vi "AlGaInPAs_v18.vi"(2 "Debug Mode":bool, 3 "Elapsed Time(s)":dbl, 4 "State":enum16{"Edit", "Start", "Run", "End", "Idle"}(ring), 5 "Argument List In":string[](array[string])) -> (0 "Status Out":string, 1 "Argument List Out":string[](array[string]))   [LabVIEW 2011]
panel:
  out "Prep-P liq var":bool
  out "P liq?":bool
  in  "Prep P liq":bool caption="Pre-run"
  in  "P Liq Flow":dbl caption="P bubbler Flow (0-100 sccm)" format="%.2f"
  in  "Run P Liq":bool caption="Run"
  out "GAMFC3 var":dbl=100.0 caption="R3 (0-1000 sscm)" format="%.1f"
  out "GAMFC2 var":dbl=10.0 caption="R2 (0-100 sscm)" format="%.2f"
  out "GAMFC1 var":dbl=1.0 caption="R1 (0-10 sscm)" format="%.2f"
  out "Ga Flow var":dbl=1.0 caption="Ga Flow (0-10 sscm)" format="%.4f"
  out "Prep-In var":bool
  out "Prep-Ga var":bool
  out "Prep-Al var":bool
  out "Prep-P gas var":bool
  out "Prep-As gas var":bool
  out "prep_done":bool
  out "run started":bool
  out "first":bool=TRUE
  out "total time":dbl
  out "is OK?":bool
  out "AsH3?":bool
  out "PH3?":bool
  out "In?":bool
  out "Ga?":bool
  out "Al?":bool
  in  "Prep As gas":bool caption="Pre-run"
  in  "Prep P gas":bool caption="Pre-run"
  in  "Prep In":bool caption="Pre-run"
  in  "prep_time":dbl caption="pre-run time (s)"
  in  "Prep Al":bool caption="Pre-run"
  in  "Run As gas":bool caption="Run"
  in  "As gas Flow":dbl caption="AsH3 Flow (0-10 sccm)" format="%.2f"
  in  "P gas Flow":dbl caption="PH3 Flow (0-100 sccm)" format="%.2f"
  in  "Run P gas":bool caption="Run"
  in  "In Flow":dbl caption="In Flow (0-100 sscm)" format="%.2f"
  in  "Run In":bool caption="Run"
  in  "Run Al":bool caption="Run"
  in  "Al Flow":dbl caption="Al Flow (0-100 sscm)" format="%.2f"
  in  "Cancel":bool
  in  "OK":bool
  out "tTotal(s) 2":dbl
  in  "Ga Tab Control":enum32{"Page 1", "Page 2", "Page 3"}(tab)
  in  "Ga Dilution":bool caption="Dilute"
  in  "Run Ga":bool caption="Run"
  in  "Prep Ga":bool caption="Pre-run"
  out "Ga Flow val":dbl=1.0 caption="Ga Flow (0-10 sscm)" format="%.4f"
  in  "Ga Flow set":dbl=1.0 caption="Ga Flow (0-10 sscm)" format="%.4f"
  out "GAMFC1 val":dbl=1.0 caption="R1 (0-10 sscm)" format="%.4f"
  out "GAMFC3 val":dbl=100.0 caption="R3 (0-1000 sscm)" format="%.1f"
  out "GAMFC2 val":dbl=10.0 caption="R2 (0-100 sscm)" format="%.2f"
  in  "GAMFC1 set":dbl=1.0 caption="R1 (0-10 sscm)" format="%.2f"
  in  "GAMFC2 set":dbl=10.0 caption="R2 (0-100 sscm)" format="%.2f"
  in  "GAMFC3 set":dbl=100.0 caption="R3 (0-1000 sscm)" format="%.1f"
  in  "Ga Calculated":u16(ring)=1 caption="Calculated" items=["Ga flow", "MFC1", "MFC2", "MFC3"]
  # "Add pre-run time to run time in editor."
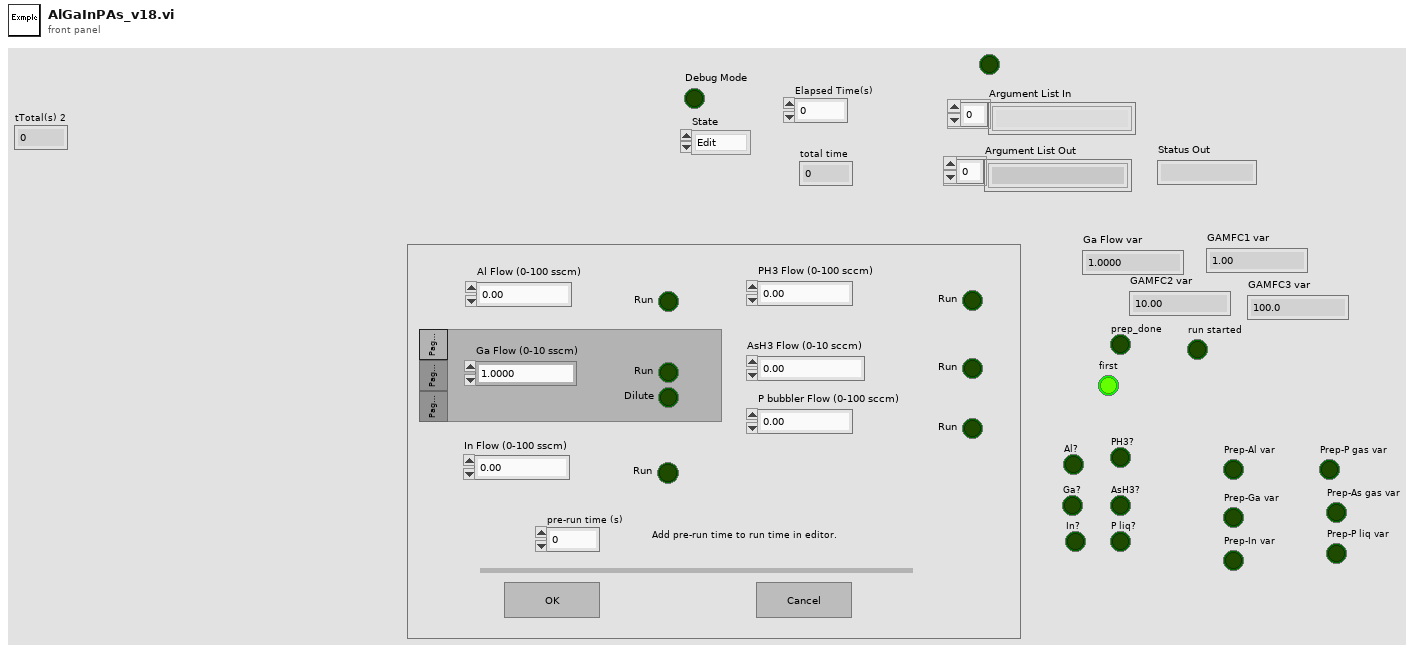
[diagram p1: front panel]
types:
  T1 = enum16{"Discrete", "Continuous", "Instantaneous", "Finite"}
  T2 = enum32{"Invalid", "Default", "Floating", "Floating/Auto-Hide", "Modal"}
  T3 = cluster{"Ga val":bool, "MFC1 val":bool, "MFC2 val":bool, "MFC3 val":bool, "Ga set":bool, "MFC1 set":bool, "MFC2 set":bool, "MFC3 set":bool}
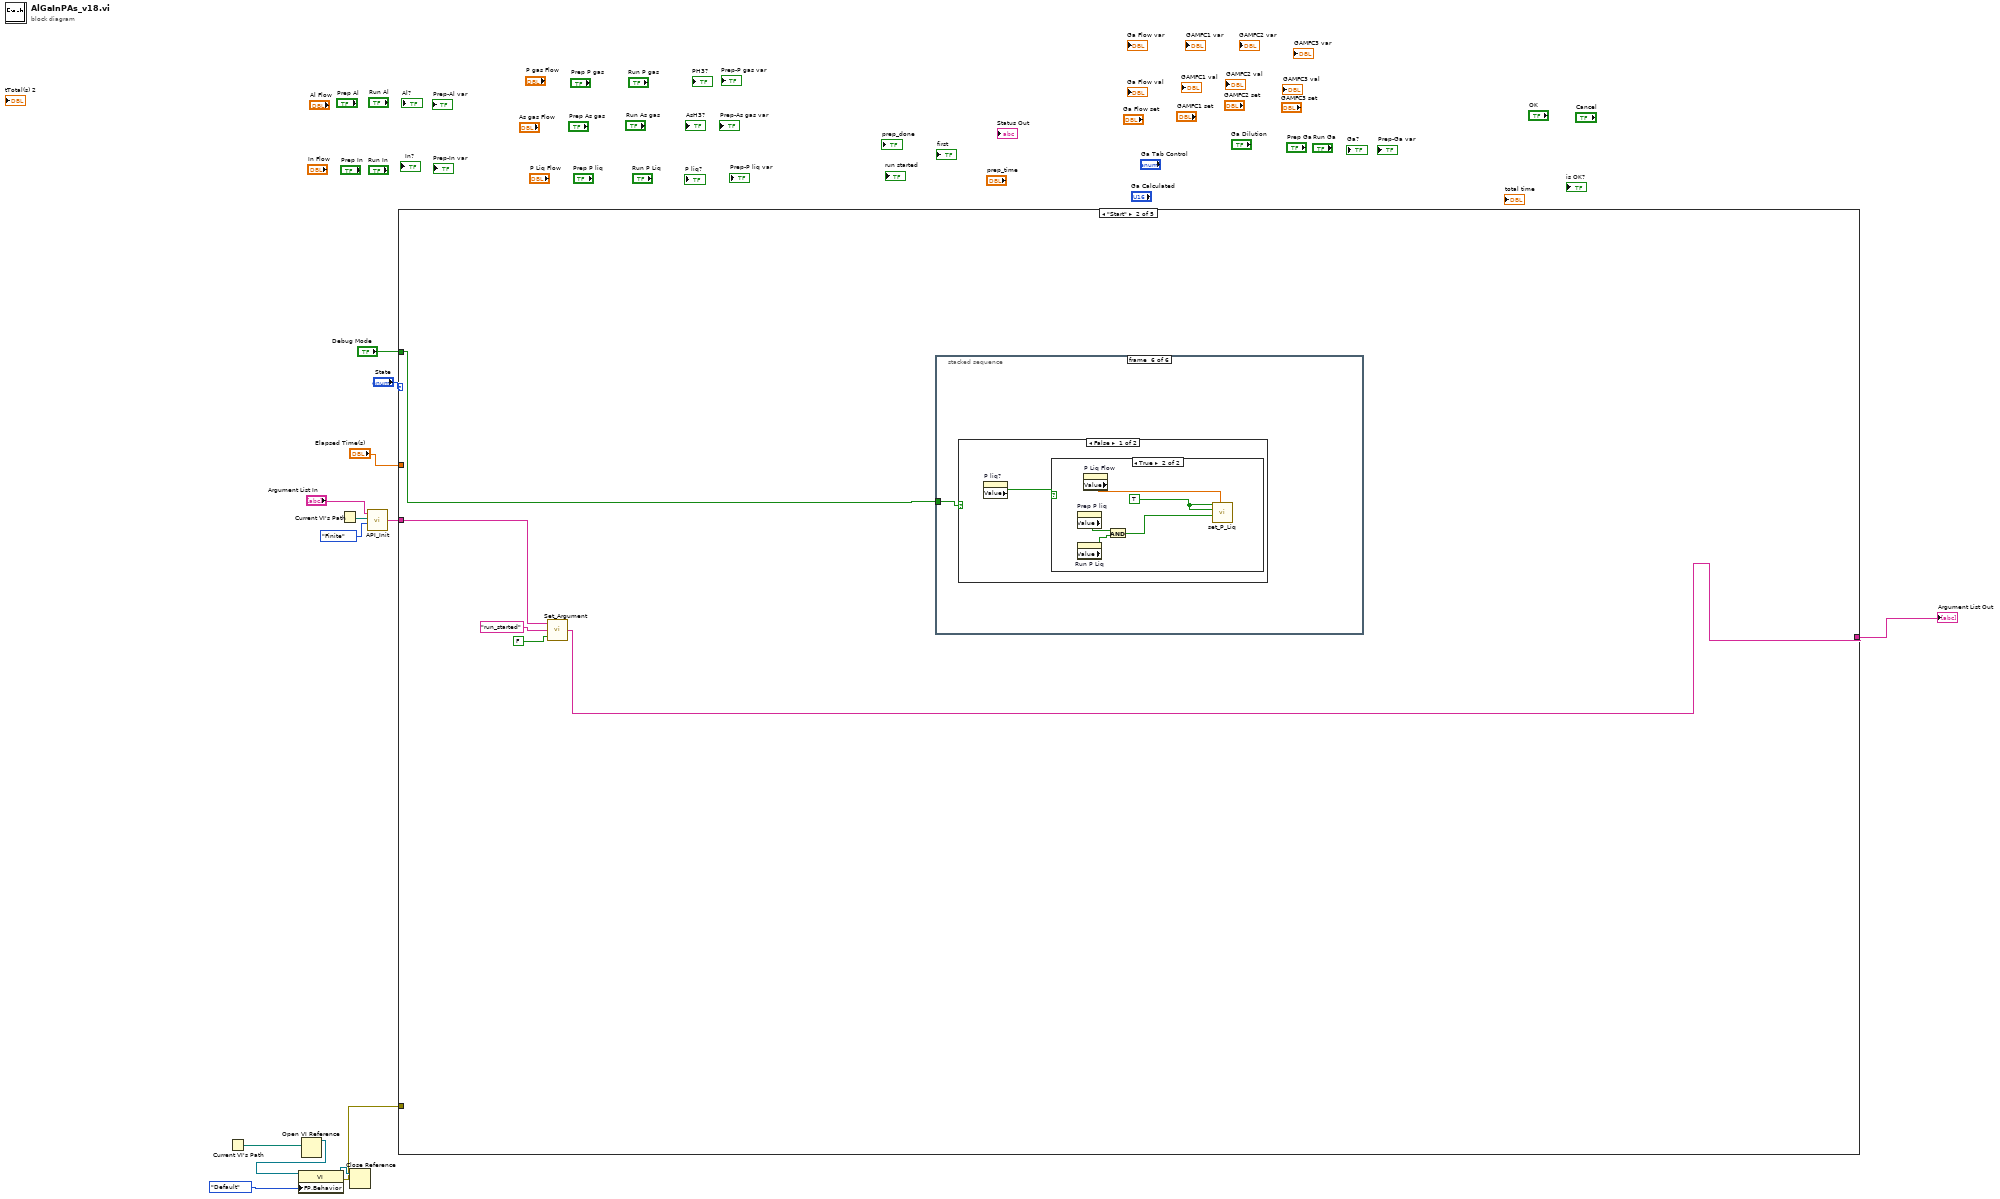
[diagram p0: block diagram]
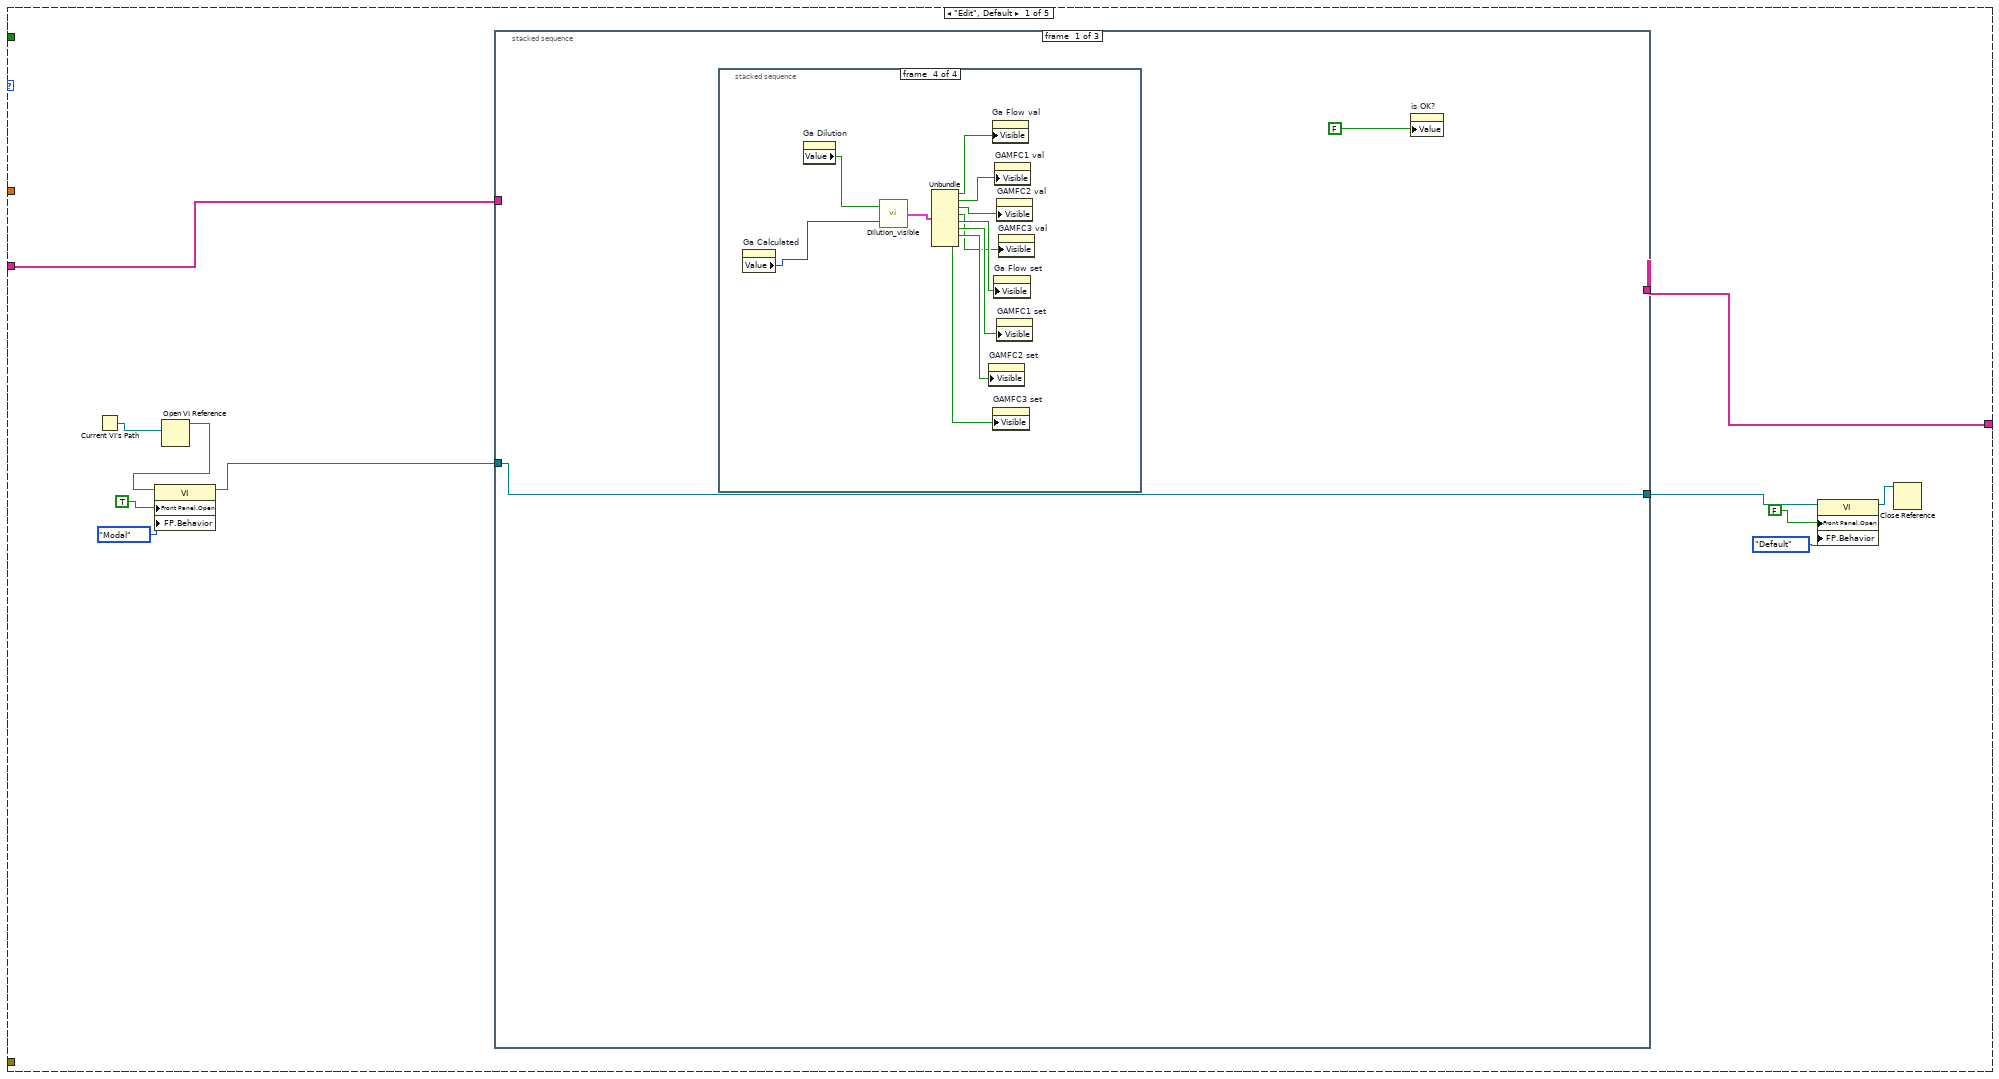
[diagram p2: hidden frame]
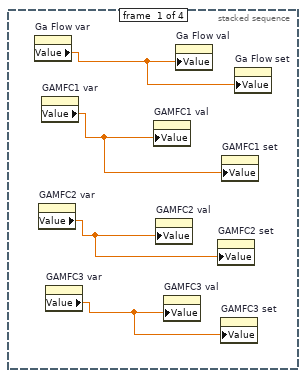
[diagram p3: hidden frame]
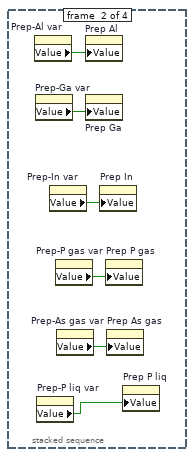
[diagram p4: hidden frame]
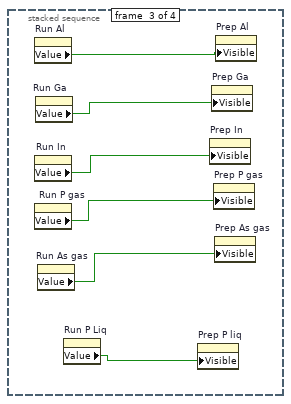
[diagram p5: hidden frame]
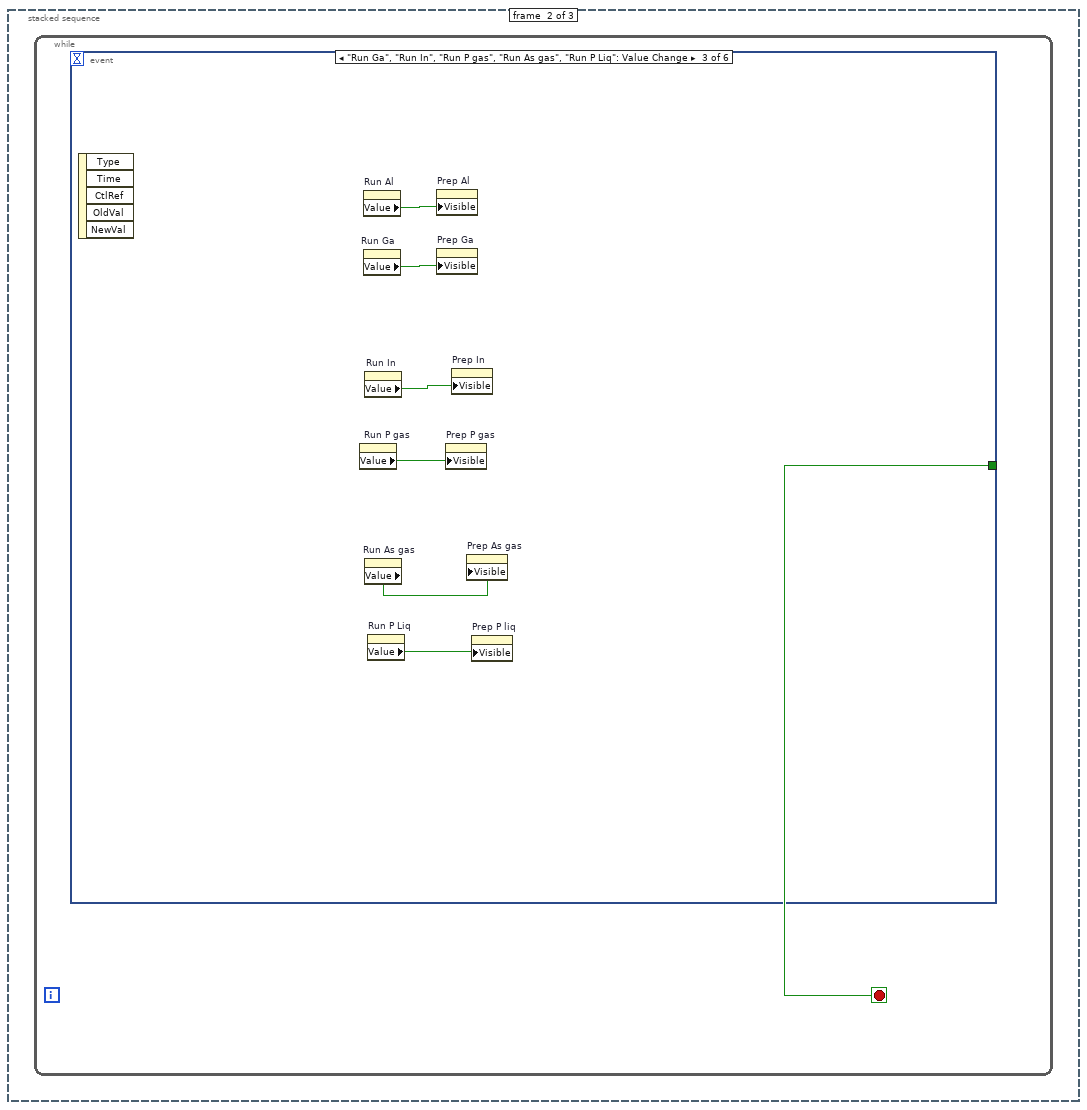
[diagram p6: hidden frame]
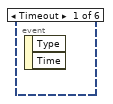
[diagram p7: hidden frame]
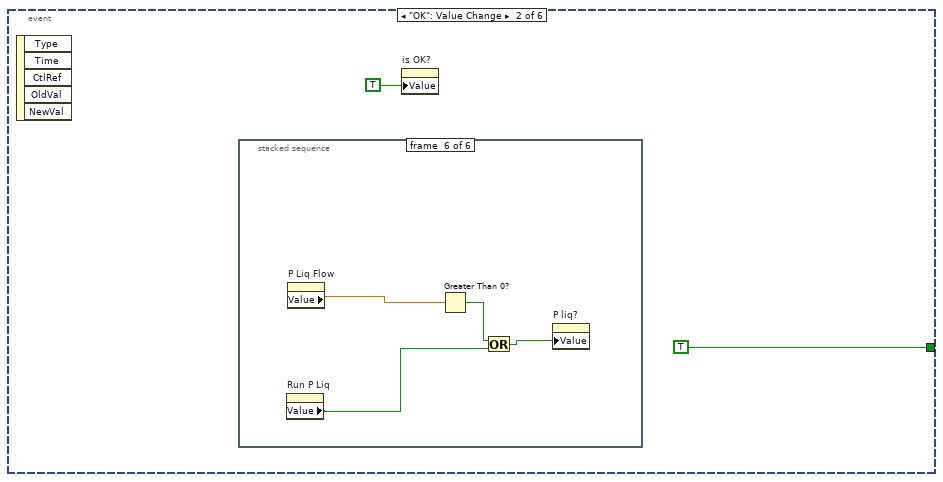
[diagram p8: hidden frame]
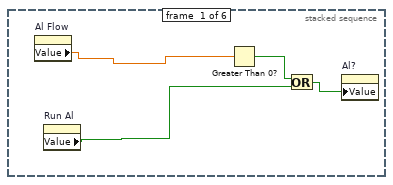
[diagram p9: hidden frame]
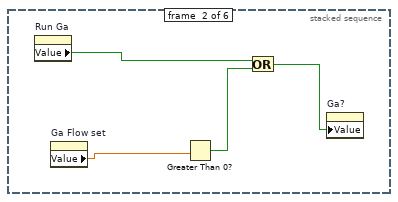
[diagram p10: hidden frame]
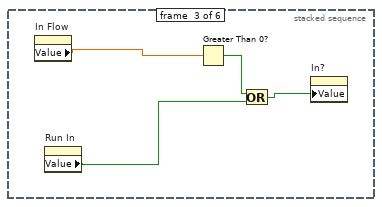
[diagram p11: hidden frame]
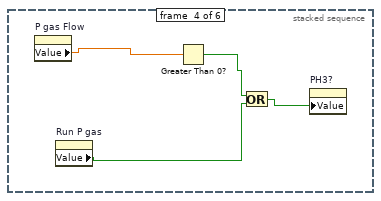
[diagram p12: hidden frame]
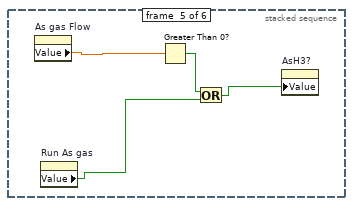
[diagram p13: hidden frame]
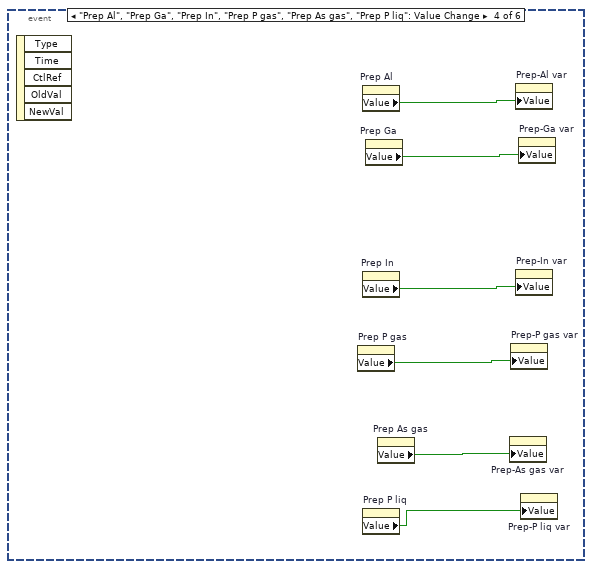
[diagram p14: hidden frame]
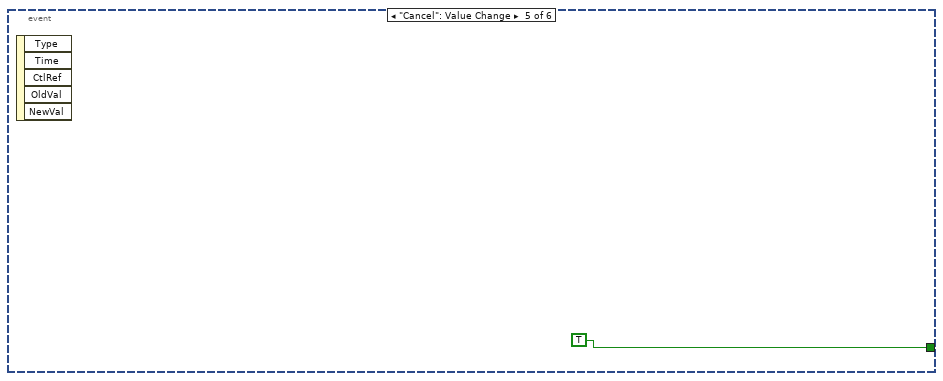
[diagram p15: hidden frame]
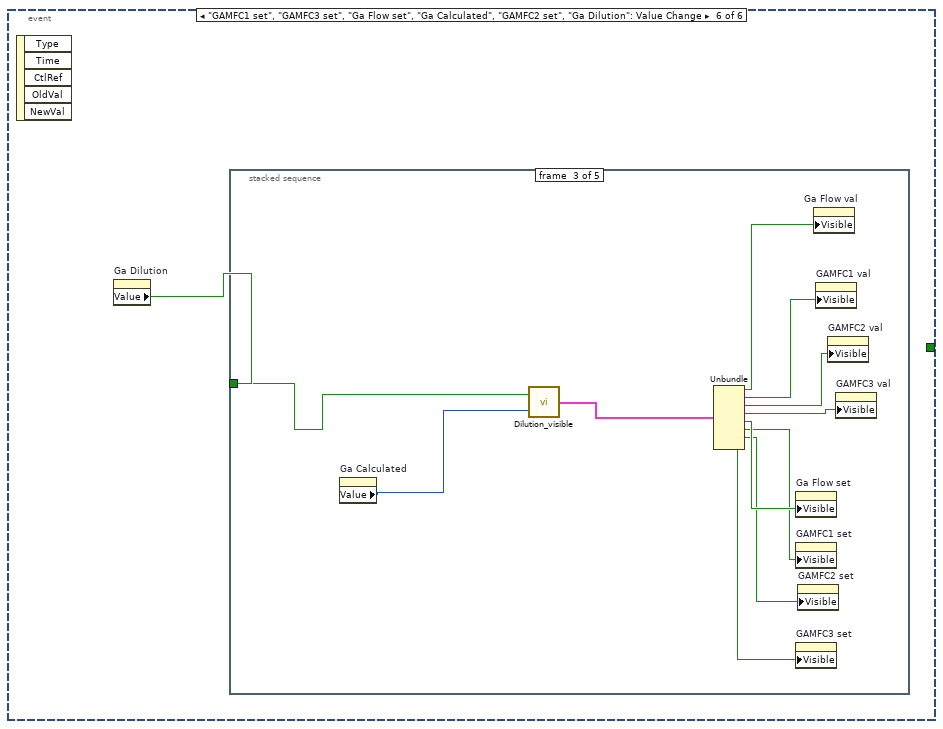
[diagram p16: hidden frame]
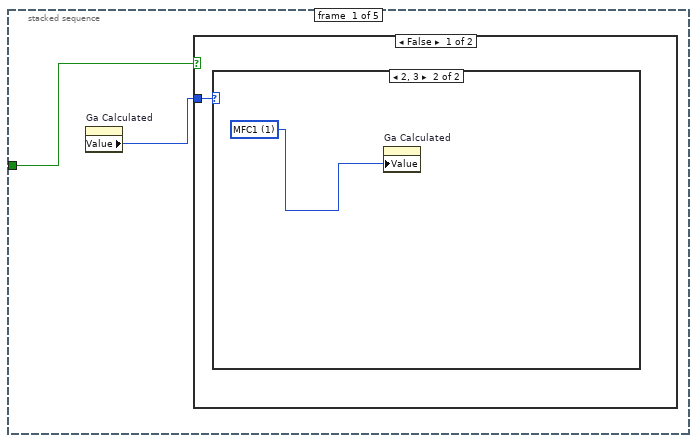
[diagram p17: hidden frame]
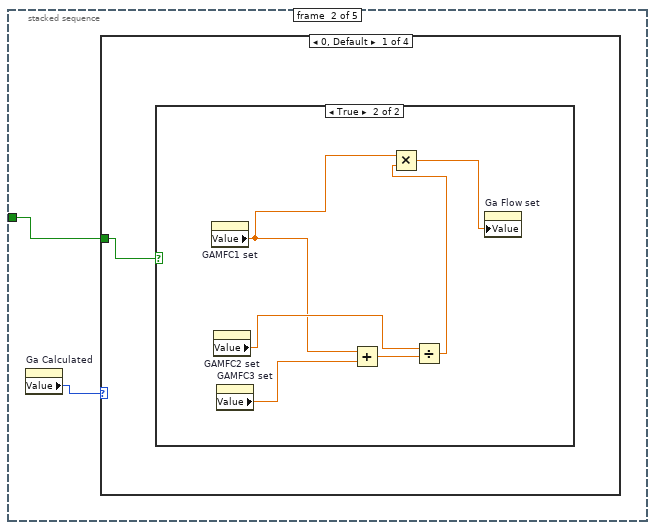
[diagram p20: hidden frame]
diagram:
  n1 = Current VI's Path() -> (path=w9:path)
  n2 = Open VI Reference(vi path=w9) -> (vi reference=w8:refnum<vi>)  [unwired: 1 in, 5 out]
  n3 = property class="VI"(reference=w8, "FP.Behavior"=T2."Default" ("Front Panel Window:Behavior")) -> (reference out=w6:refnum<vi>, error out=w5:errorcluster)  [unwired: 1 in]
  n4 = Current VI's Path() -> (path=w4:path)
  n5 = Close Reference(reference=w6) -> ()  [unwired: 1 in, 1 out]
  n6 = call "API_Init.vi"("API Mode"=T1."Finite", "VI Path"=w4, "Argument List In"="Argument List In") -> ("Argument List Out"=w1:string[])  [unwired: 1 in]
  n7 = case shown="\"Start\"" "State" {
    tunnel: "Debug Mode" -> [_ w157 w220 _ _]
    tunnel: "Elapsed Time(s)" -> [_ _ w222 _ _]
    tunnel: w1 -> [w15 w159 w219 w360 w361]
    tunnel: [w14 w158 w221 w360 w361] -> w10
    tunnel: w5 -> [_ _ _ _ _]
    frame "Edit", Default {
      n8 = Current VI's Path() -> (path=w20:path)
      n9 = Open VI Reference(vi path=w20) -> (vi reference=w19:refnum<vi>)  [unwired: 1 in, 5 out]
      n10 = property class="VI"(reference=w19, "Front Panel.Open"=TRUE ("Front Panel Window:Open"), "FP.Behavior"=T2."Modal" ("Front Panel Window:Behavior")) -> (reference out=w18:refnum<vi>)  [unwired: 1 in, 1 out]
      n11 = stacked-sequence {
        tunnel: w15 -> [_ _ w152]
        tunnel: w18 -> [w26 _ _]
        tunnel: [w26 _ _] -> w22
        tunnel: [_ _ w150] -> w14
        frame #0 {
          n12 = stacked-sequence {
            frame #0 {
              n13 = property on="Ga Flow var" class="DigNum (strict)"() -> ("Value"=w30:dbl)  [unwired: 2 in, 2 out]
              n14 = property on="GAMFC2 var" class="DigNum (strict)"() -> ("Value"=w28:dbl)  [unwired: 2 in, 2 out]
              n15 = property on="GAMFC1 var" class="DigNum (strict)"() -> ("Value"=w27:dbl)  [unwired: 2 in, 2 out]
              n16 = property on="GAMFC3 var" class="DigNum (strict)"() -> ("Value"=w29:dbl)  [unwired: 2 in, 2 out]
              n17 = property on="GAMFC1 val" class="DigNum (strict)"("Value"=w27) -> ()  [unwired: 2 in, 2 out]
              n18 = property on="GAMFC2 val" class="DigNum (strict)"("Value"=w28) -> ()  [unwired: 2 in, 2 out]
              n19 = property on="GAMFC3 val" class="DigNum (strict)"("Value"=w29) -> ()  [unwired: 2 in, 2 out]
              n20 = property on="Ga Flow val" class="DigNum (strict)"("Value"=w30) -> ()  [unwired: 2 in, 2 out]
              n21 = property on="GAMFC2 set" class="DigNum (strict)"("Value"=w28) -> ()  [unwired: 2 in, 2 out]
              n22 = property on="GAMFC3 set" class="DigNum (strict)"("Value"=w29) -> ()  [unwired: 2 in, 2 out]
              n23 = property on="GAMFC1 set" class="DigNum (strict)"("Value"=w27) -> ()  [unwired: 2 in, 2 out]
              n24 = property on="Ga Flow set" class="DigNum (strict)"("Value"=w30) -> ()  [unwired: 2 in, 2 out]
            }
            frame #1 {
              n25 = property on="Prep-Al var" class="Bool (strict)"() -> ("Value"=w36:bool)  [unwired: 2 in, 2 out]
              n26 = property on="Prep-Ga var" class="Bool (strict)"() -> ("Value"=w35:bool)  [unwired: 2 in, 2 out]
              n27 = property on="Prep-P liq var" class="Bool (strict)"() -> ("Value"=w31:bool)  [unwired: 2 in, 2 out]
              n28 = property on="Prep-In var" class="Bool (strict)"() -> ("Value"=w34:bool)  [unwired: 2 in, 2 out]
              n29 = property on="Prep-P gas var" class="Bool (strict)"() -> ("Value"=w33:bool)  [unwired: 2 in, 2 out]
              n30 = property on="Prep-As gas var" class="Bool (strict)"() -> ("Value"=w32:bool)  [unwired: 2 in, 2 out]
              n31 = property on="Prep Al" class="Bool (strict)"("Value"=w36) -> ()  [unwired: 2 in, 2 out]
              n32 = property on="Prep Ga" class="Bool (strict)"("Value"=w35) -> ()  [unwired: 2 in, 2 out]
              n33 = property on="Prep In" class="Bool (strict)"("Value"=w34) -> ()  [unwired: 2 in, 2 out]
              n34 = property on="Prep P gas" class="Bool (strict)"("Value"=w33) -> ()  [unwired: 2 in, 2 out]
              n35 = property on="Prep As gas" class="Bool (strict)"("Value"=w32) -> ()  [unwired: 2 in, 2 out]
              n36 = property on="Prep P liq" class="Bool (strict)"("Value"=w31) -> ()  [unwired: 2 in, 2 out]
            }
            frame #2 {
              n37 = property on="Run Al" class="Bool (strict)"() -> ("Value"=w42:bool)  [unwired: 2 in, 2 out]
              n38 = property on="Run In" class="Bool (strict)"() -> ("Value"=w40:bool)  [unwired: 2 in, 2 out]
              n39 = property on="Run P gas" class="Bool (strict)"() -> ("Value"=w39:bool)  [unwired: 2 in, 2 out]
              n40 = property on="Run Ga" class="Bool (strict)"() -> ("Value"=w41:bool)  [unwired: 2 in, 2 out]
              n41 = property on="Run As gas" class="Bool (strict)"() -> ("Value"=w38:bool)  [unwired: 2 in, 2 out]
              n42 = property on="Run P Liq" class="Bool (strict)"() -> ("Value"=w37:bool)  [unwired: 2 in, 2 out]
              n43 = property on="Prep P liq" class="Bool (strict)"("Visible"=w37) -> ()  [unwired: 2 in, 2 out]
              n44 = property on="Prep In" class="Bool (strict)"("Visible"=w40) -> ()  [unwired: 2 in, 2 out]
              n45 = property on="Prep Ga" class="Bool (strict)"("Visible"=w41) -> ()  [unwired: 2 in, 2 out]
              n46 = property on="Prep P gas" class="Bool (strict)"("Visible"=w39) -> ()  [unwired: 2 in, 2 out]
              n47 = property on="Prep As gas" class="Bool (strict)"("Visible"=w38) -> ()  [unwired: 2 in, 2 out]
              n48 = property on="Prep Al" class="Bool (strict)"("Visible"=w42) -> ()  [unwired: 2 in, 2 out]
            }
            frame #3 {
              n49 = property on="Ga Calculated" class="Ring (strict)"() -> ("Value"=w43:u16)  [unwired: 2 in, 2 out]
              n50 = property on="Ga Dilution" class="Bool (strict)"() -> ("Value"=w53:bool)  [unwired: 2 in, 2 out]
              n51 = call "Dilution_visible.vi"("calculated"=w43, "dilution"=w53) -> ("Visible"=w45:T3)
              n52 = Unbundle(w45) -> ("Ga val"=w46:bool, "MFC1 val"=w47:bool, "MFC2 val"=w44:bool, "MFC3 val"=w48:bool, "Ga set"=w49:bool, "MFC1 set"=w50:bool, "MFC2 set"=w51:bool, "MFC3 set"=w52:bool)
              n53 = property on="GAMFC2 set" class="DigNum (strict)"("Visible"=w51) -> ()  [unwired: 2 in, 2 out]
              n54 = property on="Ga Flow val" class="DigNum (strict)"("Visible"=w46) -> ()  [unwired: 2 in, 2 out]
              n55 = property on="GAMFC3 set" class="DigNum (strict)"("Visible"=w52) -> ()  [unwired: 2 in, 2 out]
              n56 = property on="Ga Flow set" class="DigNum (strict)"("Visible"=w49) -> ()  [unwired: 2 in, 2 out]
              n57 = property on="GAMFC1 val" class="DigNum (strict)"("Visible"=w47) -> ()  [unwired: 2 in, 2 out]
              n58 = property on="GAMFC2 val" class="DigNum (strict)"("Visible"=w44) -> ()  [unwired: 2 in, 2 out]
              n59 = property on="GAMFC1 set" class="DigNum (strict)"("Visible"=w50) -> ()  [unwired: 2 in, 2 out]
              n60 = property on="GAMFC3 val" class="DigNum (strict)"("Visible"=w48) -> ()  [unwired: 2 in, 2 out]
            }
          }
          n61 = property on="is OK?" class="Bool (strict)"("Value"=FALSE ("is OK?")) -> ()  [unwired: 2 in, 2 out]
        }
        frame #1 {
          n62 = while {
            stop <- w54 stop-if-true
            n63 = event shown="[2] \"Run Ga\", \"Run In\", \"Run P gas\", \"Run As gas\", \"Run P Liq\": Value Change" {
              selector: _ -> [_ _ _ _ _ _]
              dyn-events: _ -> [_ _ _ _ _ _]
              timeout: _ -> [_ _ _ _ _ _]
              tunnel: [_ TRUE _ _ TRUE _] -> w54
              event Timeout {
                n64 = event-data() -> ()  [unwired: 1 in, 2 out]
              }
              event "OK": Value Change {
                n65 = event-data() -> ()  [unwired: 1 in, 5 out]
                n66 = stacked-sequence {
                  frame #0 {
                    n67 = property on="Al Flow" class="DigNum (strict)"() -> ("Value"=w59:dbl)  [unwired: 2 in, 2 out]
                    n68 = property on="Run Al" class="Bool (strict)"() -> ("Value"=w58:bool)  [unwired: 2 in, 2 out]
                    n69 = Greater Than 0?(x=w59) -> (x > 0?=w60:bool)
                    n70 = Or(x=w60, y=w58) -> (x .or. y?=w57:bool)
                    n71 = property on="Al?" class="Bool (strict)"("Value"=w57) -> ()  [unwired: 2 in, 2 out]
                  }
                  frame #1 {
                    n72 = property on="Run Ga" class="Bool (strict)"() -> ("Value"=w62:bool)  [unwired: 2 in, 2 out]
                    n73 = property on="Ga Flow set" class="DigNum (strict)"() -> ("Value"=w63:dbl)  [unwired: 2 in, 2 out]
                    n74 = Greater Than 0?(x=w63) -> (x > 0?=w64:bool)
                    n75 = Or(x=w62, y=w64) -> (x .or. y?=w61:bool)
                    n76 = property on="Ga?" class="Bool (strict)"("Value"=w61) -> ()  [unwired: 2 in, 2 out]
                  }
                  frame #2 {
                    n77 = property on="In Flow" class="DigNum (strict)"() -> ("Value"=w66:dbl)  [unwired: 2 in, 2 out]
                    n78 = property on="Run In" class="Bool (strict)"() -> ("Value"=w67:bool)  [unwired: 2 in, 2 out]
                    n79 = Greater Than 0?(x=w66) -> (x > 0?=w68:bool)
                    n80 = Or(x=w68, y=w67) -> (x .or. y?=w65:bool)
                    n81 = property on="In?" class="Bool (strict)"("Value"=w65) -> ()  [unwired: 2 in, 2 out]
                  }
                  frame #3 {
                    n82 = property on="P gas Flow" class="DigNum (strict)"() -> ("Value"=w71:dbl)  [unwired: 2 in, 2 out]
                    n83 = property on="Run P gas" class="Bool (strict)"() -> ("Value"=w70:bool)  [unwired: 2 in, 2 out]
                    n84 = Greater Than 0?(x=w71) -> (x > 0?=w72:bool)
                    n85 = Or(x=w72, y=w70) -> (x .or. y?=w69:bool)
                    n86 = property on="PH3?" class="Bool (strict)"("Value"=w69) -> ()  [unwired: 2 in, 2 out]
                  }
                  frame #4 {
                    n87 = property on="As gas Flow" class="DigNum (strict)"() -> ("Value"=w75:dbl)  [unwired: 2 in, 2 out]
                    n88 = property on="Run As gas" class="Bool (strict)"() -> ("Value"=w74:bool)  [unwired: 2 in, 2 out]
                    n89 = Greater Than 0?(x=w75) -> (x > 0?=w76:bool)
                    n90 = Or(x=w76, y=w74) -> (x .or. y?=w73:bool)
                    n91 = property on="AsH3?" class="Bool (strict)"("Value"=w73) -> ()  [unwired: 2 in, 2 out]
                  }
                  frame #5 {
                    n92 = property on="Run P Liq" class="Bool (strict)"() -> ("Value"=w79:bool)  [unwired: 2 in, 2 out]
                    n93 = property on="P Liq Flow" class="DigNum (strict)"() -> ("Value"=w78:dbl)  [unwired: 2 in, 2 out]
                    n94 = Greater Than 0?(x=w78) -> (x > 0?=w80:bool)
                    n95 = Or(x=w80, y=w79) -> (x .or. y?=w77:bool)
                    n96 = property on="P liq?" class="Bool (strict)"("Value"=w77) -> ()  [unwired: 2 in, 2 out]
                  }
                }
                n97 = property on="is OK?" class="Bool (strict)"("Value"=TRUE ("is OK?")) -> ()  [unwired: 2 in, 2 out]
              }
              event "Run Ga", "Run In", "Run P gas", "Run As gas", "Run P Liq": Value Change {
                n98 = event-data() -> ()  [unwired: 1 in, 5 out]
                n99 = property on="Run P gas" class="Bool (strict)"() -> ("Value"=w82:bool)  [unwired: 2 in, 2 out]
                n100 = property on="Run Al" class="Bool (strict)"() -> ("Value"=w86:bool)  [unwired: 2 in, 2 out]
                n101 = property on="Run Ga" class="Bool (strict)"() -> ("Value"=w85:bool)  [unwired: 2 in, 2 out]
                n102 = property on="Run In" class="Bool (strict)"() -> ("Value"=w84:bool)  [unwired: 2 in, 2 out]
                n103 = property on="Run As gas" class="Bool (strict)"() -> ("Value"=w83:bool)  [unwired: 2 in, 2 out]
                n104 = property on="Run P Liq" class="Bool (strict)"() -> ("Value"=w81:bool)  [unwired: 2 in, 2 out]
                n105 = property on="Prep Al" class="Bool (strict)"("Visible"=w86) -> ()  [unwired: 2 in, 2 out]
                n106 = property on="Prep Ga" class="Bool (strict)"("Visible"=w85) -> ()  [unwired: 2 in, 2 out]
                n107 = property on="Prep P gas" class="Bool (strict)"("Visible"=w82) -> ()  [unwired: 2 in, 2 out]
                n108 = property on="Prep In" class="Bool (strict)"("Visible"=w84) -> ()  [unwired: 2 in, 2 out]
                n109 = property on="Prep As gas" class="Bool (strict)"("Visible"=w83) -> ()  [unwired: 2 in, 2 out]
                n110 = property on="Prep P liq" class="Bool (strict)"("Visible"=w81) -> ()  [unwired: 2 in, 2 out]
              }
              event "Prep Al", "Prep Ga", "Prep In", "Prep P gas", "Prep As gas", "Prep P liq": Value Change {
                n111 = event-data() -> ()  [unwired: 1 in, 5 out]
                n112 = property on="Prep P gas" class="Bool (strict)"() -> ("Value"=w89:bool)  [unwired: 2 in, 2 out]
                n113 = property on="Prep Al" class="Bool (strict)"() -> ("Value"=w92:bool)  [unwired: 2 in, 2 out]
                n114 = property on="Prep In" class="Bool (strict)"() -> ("Value"=w90:bool)  [unwired: 2 in, 2 out]
                n115 = property on="Prep P liq" class="Bool (strict)"() -> ("Value"=w87:bool)  [unwired: 2 in, 2 out]
                n116 = property on="Prep Ga" class="Bool (strict)"() -> ("Value"=w91:bool)  [unwired: 2 in, 2 out]
                n117 = property on="Prep As gas" class="Bool (strict)"() -> ("Value"=w88:bool)  [unwired: 2 in, 2 out]
                n118 = property on="Prep-As gas var" class="Bool (strict)"("Value"=w88) -> ()  [unwired: 2 in, 2 out]
                n119 = property on="Prep-P gas var" class="Bool (strict)"("Value"=w89) -> ()  [unwired: 2 in, 2 out]
                n120 = property on="Prep-Al var" class="Bool (strict)"("Value"=w92) -> ()  [unwired: 2 in, 2 out]
                n121 = property on="Prep-In var" class="Bool (strict)"("Value"=w90) -> ()  [unwired: 2 in, 2 out]
                n122 = property on="Prep-Ga var" class="Bool (strict)"("Value"=w91) -> ()  [unwired: 2 in, 2 out]
                n123 = property on="Prep-P liq var" class="Bool (strict)"("Value"=w87) -> ()  [unwired: 2 in, 2 out]
              }
              event "Cancel": Value Change {
                n124 = event-data() -> ()  [unwired: 1 in, 5 out]
              }
              event "GAMFC1 set", "GAMFC3 set", "Ga Flow set", "Ga Calculated", "GAMFC2 set", "Ga Dilution": Value Change {
                n125 = event-data() -> ()  [unwired: 1 in, 5 out]
                n126 = property on="Ga Dilution" class="Bool (strict)"() -> ("Value"=w94:bool)  [unwired: 2 in, 2 out]
                n127 = stacked-sequence {
                  tunnel: w94 -> [w96 w100 w141 _ w146]
                  frame #0 {
                    n128 = property on="Ga Calculated" class="Ring (strict)"() -> ("Value"=w95:u16)  [unwired: 2 in, 2 out]
                    n129 = case shown="False" w96 {
                      tunnel: w95 -> [w97 _]
                      frame False {
                        n130 = case shown="2, 3" w97 {
                          frame 0, 1, Default {
                          }
                          frame 2, 3 {
                            w98 = u16 1 items=["Ga flow", "MFC1", "MFC2", "MFC3"] ("Ga calculated")
                            n131 = property on="Ga Calculated" class="Ring (strict)"("Value"=w98) -> ()  [unwired: 2 in, 2 out]
                          }
                        }
                      }
                      frame True {
                      }
                    }
                  }
                  frame #1 {
                    n132 = property on="Ga Calculated" class="Ring (strict)"() -> ("Value"=w99:u16)  [unwired: 2 in, 2 out]
                    n133 = case shown="0, Default" w99 {
                      tunnel: w100 -> [w101 w109 w117 w124]
                      frame 0, Default {
                        n134 = case shown="True" w101 {
                          frame False {
                            n135 = property on="GAMFC1 set" class="DigNum (strict)"() -> ("Value"=w102:dbl)  [unwired: 2 in, 2 out]
                            n136 = property on="Ga Flow set" class="DigNum (strict)"("Value"=w102) -> ()  [unwired: 2 in, 2 out]
                          }
                          frame True {
                            n137 = property on="GAMFC1 set" class="DigNum (strict)"() -> ("Value"=w104:dbl)  [unwired: 2 in, 2 out]
                            n138 = property on="GAMFC2 set" class="DigNum (strict)"() -> ("Value"=w106:dbl)  [unwired: 2 in, 2 out]
                            n139 = property on="GAMFC3 set" class="DigNum (strict)"() -> ("Value"=w108:dbl)  [unwired: 2 in, 2 out]
                            n140 = Add(x=w104, y=w108) -> (x+y=w107:dbl)
                            n141 = Divide(x=w106, y=w107) -> (x/y=w105:dbl)
                            n142 = Multiply(x=w104, y=w105) -> (x*y=w103:dbl)
                            n143 = property on="Ga Flow set" class="DigNum (strict)"("Value"=w103) -> ()  [unwired: 2 in, 2 out]
                          }
                        }
                      }
                      frame 1 {
                        n144 = case shown="True" w109 {
                          frame False {
                            n145 = property on="Ga Flow set" class="DigNum (strict)"() -> ("Value"=w110:dbl)  [unwired: 2 in, 2 out]
                            n146 = property on="GAMFC1 set" class="DigNum (strict)"("Value"=w110) -> ()  [unwired: 2 in, 2 out]
                          }
                          frame True {
                            n147 = property on="Ga Flow set" class="DigNum (strict)"() -> ("Value"=w115:dbl)  [unwired: 2 in, 2 out]
                            n148 = property on="GAMFC2 set" class="DigNum (strict)"() -> ("Value"=w116:dbl)  [unwired: 2 in, 2 out]
                            n149 = property on="GAMFC3 set" class="DigNum (strict)"() -> ("Value"=w114:dbl)  [unwired: 2 in, 2 out]
                            n150 = Subtract(x=w116, y=w115) -> (x-y=w112:dbl)
                            n151 = Multiply(x=w115, y=w114) -> (x*y=w113:dbl)
                            n152 = Divide(x=w113, y=w112) -> (x/y=w111:dbl)
                            n153 = property on="GAMFC1 set" class="DigNum (strict)"("Value"=w111) -> ()  [unwired: 2 in, 2 out]
                          }
                        }
                      }
                      frame 2 {
                        n154 = case shown="True" w117 {
                          frame False {
                          }
                          frame True {
                            n155 = property on="GAMFC1 set" class="DigNum (strict)"() -> ("Value"=w119:dbl)  [unwired: 2 in, 2 out]
                            n156 = property on="GAMFC3 set" class="DigNum (strict)"() -> ("Value"=w121:dbl)  [unwired: 2 in, 2 out]
                            n157 = property on="Ga Flow set" class="DigNum (strict)"() -> ("Value"=w122:dbl)  [unwired: 2 in, 2 out]
                            n158 = Add(x=w119, y=w121) -> (x+y=w123:dbl)
                            n159 = Multiply(x=w122, y=w123) -> (x*y=w120:dbl)
                            n160 = Divide(x=w120, y=w119) -> (x/y=w118:dbl)
                            n161 = property on="GAMFC2 set" class="DigNum (strict)"("Value"=w118) -> ()  [unwired: 2 in, 2 out]
                          }
                        }
                      }
                      frame 3 {
                        n162 = case shown="True" w124 {
                          frame False {
                          }
                          frame True {
                            n163 = property on="GAMFC2 set" class="DigNum (strict)"() -> ("Value"=w130:dbl)  [unwired: 2 in, 2 out]
                            n164 = property on="Ga Flow set" class="DigNum (strict)"() -> ("Value"=w128:dbl)  [unwired: 2 in, 2 out]
                            n165 = property on="GAMFC1 set" class="DigNum (strict)"() -> ("Value"=w129:dbl)  [unwired: 2 in, 2 out]
                            n166 = Subtract(x=w130, y=w128) -> (x-y=w126:dbl)
                            n167 = Divide(x=w129, y=w128) -> (x/y=w127:dbl)
                            n168 = Multiply(x=w127, y=w126) -> (x*y=w125:dbl)
                            n169 = property on="GAMFC3 set" class="DigNum (strict)"("Value"=w125) -> ()  [unwired: 2 in, 2 out]
                          }
                        }
                      }
                    }
                  }
                  frame #2 {
                    n170 = property on="Ga Calculated" class="Ring (strict)"() -> ("Value"=w131:u16)  [unwired: 2 in, 2 out]
                    n171 = call "Dilution_visible.vi"("calculated"=w131, "dilution"=w141) -> ("Visible"=w137:T3)
                    n172 = Unbundle(w137) -> ("Ga val"=w140:bool, "MFC1 val"=w139:bool, "MFC2 val"=w138:bool, "MFC3 val"=w136:bool, "Ga set"=w135:bool, "MFC1 set"=w134:bool, "MFC2 set"=w133:bool, "MFC3 set"=w132:bool)
                    n173 = property on="Ga Flow set" class="DigNum (strict)"("Visible"=w135) -> ()  [unwired: 2 in, 2 out]
                    n174 = property on="GAMFC1 set" class="DigNum (strict)"("Visible"=w134) -> ()  [unwired: 2 in, 2 out]
                    n175 = property on="GAMFC3 set" class="DigNum (strict)"("Visible"=w132) -> ()  [unwired: 2 in, 2 out]
                    n176 = property on="GAMFC2 set" class="DigNum (strict)"("Visible"=w133) -> ()  [unwired: 2 in, 2 out]
                    n177 = property on="Ga Flow val" class="DigNum (strict)"("Visible"=w140) -> ()  [unwired: 2 in, 2 out]
                    n178 = property on="GAMFC1 val" class="DigNum (strict)"("Visible"=w139) -> ()  [unwired: 2 in, 2 out]
                    n179 = property on="GAMFC2 val" class="DigNum (strict)"("Visible"=w138) -> ()  [unwired: 2 in, 2 out]
                    n180 = property on="GAMFC3 val" class="DigNum (strict)"("Visible"=w136) -> ()  [unwired: 2 in, 2 out]
                  }
                  frame #3 {
                    n181 = property on="GAMFC1 set" class="DigNum (strict)"() -> ("Value"=w144:dbl)  [unwired: 2 in, 2 out]
                    n182 = property on="Ga Flow set" class="DigNum (strict)"() -> ("Value"=w145:dbl)  [unwired: 2 in, 2 out]
                    n183 = property on="GAMFC2 set" class="DigNum (strict)"() -> ("Value"=w143:dbl)  [unwired: 2 in, 2 out]
                    n184 = property on="GAMFC3 set" class="DigNum (strict)"() -> ("Value"=w142:dbl)  [unwired: 2 in, 2 out]
                    n185 = property on="GAMFC3 val" class="DigNum (strict)"("Value"=w142) -> ()  [unwired: 2 in, 2 out]
                    n186 = property on="GAMFC1 val" class="DigNum (strict)"("Value"=w144) -> ()  [unwired: 2 in, 2 out]
                    n187 = property on="GAMFC2 val" class="DigNum (strict)"("Value"=w143) -> ()  [unwired: 2 in, 2 out]
                    n188 = property on="Ga Flow val" class="DigNum (strict)"("Value"=w145) -> ()  [unwired: 2 in, 2 out]
                    n189 = property on="GAMFC3 var" class="DigNum (strict)"("Value"=w142) -> ()  [unwired: 2 in, 2 out]
                    n190 = property on="GAMFC1 var" class="DigNum (strict)"("Value"=w144) -> ()  [unwired: 2 in, 2 out]
                    n191 = property on="GAMFC2 var" class="DigNum (strict)"("Value"=w143) -> ()  [unwired: 2 in, 2 out]
                    n192 = property on="Ga Flow var" class="DigNum (strict)"("Value"=w145) -> ()  [unwired: 2 in, 2 out]
                  }
                  frame #4 {
                    n193 = case shown="True" w146 {
                      frame False {
                        n194 = property on="Ga Calculated" class="Ring (strict)"("Disabled Items []"=i32[] [2, 3]) -> ()  [unwired: 2 in, 2 out]
                      }
                      frame True {
                        n195 = property on="Ga Calculated" class="Ring (strict)"("Disabled Items []"=i32[] []) -> ()  [unwired: 2 in, 2 out]
                      }
                    }
                  }
                }
              }
            }
          }
        }
        frame #2 {
          n196 = property on="is OK?" class="Bool (strict)"() -> ("Value"=w149:bool)  [unwired: 2 in, 2 out]
          n197 = case shown="True" w149 {
            tunnel: w152 -> [w155 w156]
            tunnel: [w155 w156] -> w151
            frame False {
            }
            frame True {
            }
          }
          n198 = Not(x=w149) -> (.not. x?=w154:bool)
          n199 = Current VI's Path() -> (path=w153:path)
          n200 = call "API_Edit.vi"("Cancel"=w154, "OK"=w149, "VI Path"=w153, "Argument List In"=w151) -> ("Argument List Out"=w150:string[])
        }
      }
      n201 = property class="VI"(reference=w22, "Front Panel.Open"=FALSE ("Front Panel Window:Open"), "FP.Behavior"=T2."Default" ("Front Panel Window:Behavior")) -> (reference out=w23:refnum<vi>)  [unwired: 1 in, 1 out]
      n202 = Close Reference(reference=w23) -> ()  [unwired: 1 in, 1 out]
    }
    frame "Start" {
      n203 = call "Set_Argument.vi"("Enable"=FALSE, "Argument"="run_started", "Argument List In"=w159) -> ("Argument List Out"=w158:string[])
      n204 = stacked-sequence {
        tunnel: w157 -> [w162 w171 w183 w192 w201 w210]
        frame #0 {
          n205 = case shown="False" w162 {
            frame False {
              n206 = property on="Al?" class="Bool (strict)"() -> ("Value"=w163:bool)  [unwired: 2 in, 2 out]
              n207 = case shown="True" w163 {
                frame False {
                  w164 = FALSE ("Al Active")
                  n208 = call "set_Al.vi"("ALMFC1"=0.0 ("Aluminum Flow"), "Remote"=w164, "Run"=w164, "Bubbler In"=w164, "Active"=w164) -> ()  [unwired: 5 out]
                }
                frame True {
                  w170 = TRUE ("Al Active")
                  n209 = property on="Prep Al" class="Bool (strict)"() -> ("Value"=w168:bool)  [unwired: 2 in, 2 out]
                  n210 = property on="Run Al" class="Bool (strict)"() -> ("Value"=w167:bool)  [unwired: 2 in, 2 out]
                  n211 = property on="Al Flow" class="DigNum (strict)"() -> ("Value"=w169:dbl)  [unwired: 2 in, 2 out]
                  n212 = And(x=w168, y=w167) -> (x .and. y?=w166:bool)
                  n213 = call "set_Al.vi"("ALMFC1"=w169, "Run"=w166, "Bubbler In"=w170, "Active"=w170) -> ()  [unwired: 1 in, 5 out]
                }
              }
            }
            frame True {
            }
          }
        }
        frame #1 {
          n214 = case shown="False" w171 {
            frame False {
              n215 = property on="Ga?" class="Bool (strict)"() -> ("Value"=w172:bool)  [unwired: 2 in, 2 out]
              n216 = case shown="True" w172 {
                frame False {
                  w174 = FALSE ("Ga Active")
                  w173 = 0.0 ("Ga Flow 1")
                  n217 = call "set_Ga.vi"("Active"=w174, "GAMFC3"=w173, "GAMFC2"=w173, "GAMFC1"=w173, "Bubbler In"=w174, "H2 Dilute"=w174, "Run"=w174, "Remote"=w174) -> ()  [unwired: 8 out]
                }
                frame True {
                  w178 = TRUE ("Ga Active")
                  n218 = property on="GAMFC3 var" class="DigNum (strict)"() -> ("Value"=w175:dbl)  [unwired: 2 in, 2 out]
                  n219 = property on="GAMFC2 var" class="DigNum (strict)"() -> ("Value"=w176:dbl)  [unwired: 2 in, 2 out]
                  n220 = property on="GAMFC1 var" class="DigNum (strict)"() -> ("Value"=w177:dbl)  [unwired: 2 in, 2 out]
                  n221 = property on="Prep-Ga var" class="Bool (strict)"() -> ("Value"=w179:bool)  [unwired: 2 in, 2 out]
                  n222 = property on="Run Ga" class="Bool (strict)"() -> ("Value"=w180:bool)  [unwired: 2 in, 2 out]
                  n223 = And(x=w179, y=w180) -> (x .and. y?=w182:bool)
                  n224 = property on="Ga Dilution" class="Bool (strict)"() -> ("Value"=w181:bool)  [unwired: 2 in, 2 out]
                  n225 = call "set_Ga.vi"("Active"=w178, "GAMFC3"=w175, "GAMFC2"=w176, "GAMFC1"=w177, "Bubbler In"=w178, "H2 Dilute"=w181, "Run"=w182, "Remote"=w178) -> ()  [unwired: 8 in]
                }
              }
            }
            frame True {
            }
          }
        }
        frame #2 {
          n226 = case shown="False" w183 {
            frame False {
              n227 = property on="In?" class="Bool (strict)"() -> ("Value"=w184:bool)  [unwired: 2 in, 2 out]
              n228 = case shown="True" w184 {
                frame False {
                  w186 = FALSE ("In Remote")
                  n229 = call "set_In.vi"("INMFC1"=0.0 ("Indium Flow"), "Remote"=w186, "Run"=w186, "Bubbler In"=w186, "Active"=w186) -> ()  [unwired: 5 out]
                }
                frame True {
                  w191 = TRUE ("In Run")
                  n230 = property on="Run In" class="Bool (strict)"() -> ("Value"=w188:bool)  [unwired: 2 in, 2 out]
                  n231 = property on="Prep In" class="Bool (strict)"() -> ("Value"=w189:bool)  [unwired: 2 in, 2 out]
                  n232 = And(x=w189, y=w188) -> (x .and. y?=w187:bool)
                  n233 = property on="In Flow" class="DigNum (strict)"() -> ("Value"=w190:dbl)  [unwired: 2 in, 2 out]
                  n234 = call "set_In.vi"("INMFC1"=w190, "Run"=w187, "Bubbler In"=w191, "Active"=w191) -> ()  [unwired: 1 in, 5 out]
                }
              }
            }
            frame True {
            }
          }
        }
        frame #3 {
          n235 = case shown="False" w192 {
            frame False {
              n236 = property on="PH3?" class="Bool (strict)"() -> ("Value"=w193:bool)  [unwired: 2 in, 2 out]
              n237 = case shown="True" w193 {
                frame False {
                  w194 = FALSE ("P_Gas Active")
                  n238 = call "set_P_gas.vi"("Run"=w194, "Gas In"=w194, "Active"=w194, "P_Gas Remote"=w194, "H2 Flush"=w194, "P_Gas Flow"=0.0) -> ()
                }
                frame True {
                  w200 = TRUE ("P_Gas Active")
                  n239 = property on="P gas Flow" class="DigNum (strict)"() -> ("Value"=w199:dbl)  [unwired: 2 in, 2 out]
                  n240 = property on="Prep P gas" class="Bool (strict)"() -> ("Value"=w198:bool)  [unwired: 2 in, 2 out]
                  n241 = property on="Run P gas" class="Bool (strict)"() -> ("Value"=w197:bool)  [unwired: 2 in, 2 out]
                  n242 = And(x=w198, y=w197) -> (x .and. y?=w196:bool)
                  n243 = call "set_P_gas.vi"("Active"=w200, "P_Gas Remote"=w196, "H2 Flush"=w200, "P_Gas Flow"=w199) -> ()  [unwired: 2 in]
                }
              }
            }
            frame True {
            }
          }
        }
        frame #4 {
          n244 = case shown="False" w201 {
            frame False {
              n245 = property on="AsH3?" class="Bool (strict)"() -> ("Value"=w202:bool)  [unwired: 2 in, 2 out]
              n246 = case shown="True" w202 {
                frame False {
                  w203 = FALSE ("As_Gas Active")
                  n247 = call "set_As_gas.vi"("Active"=w203, "As_Gas Flow"=0.0, "Gas In"=w203, "H2 Flush"=w203, "Run"=w203, "Remote"=w203) -> ()  [unwired: 10 in]
                }
                frame True {
                  w209 = TRUE ("As_Gas Active")
                  n248 = property on="Prep As gas" class="Bool (strict)"() -> ("Value"=w206:bool)  [unwired: 2 in, 2 out]
                  n249 = property on="Run As gas" class="Bool (strict)"() -> ("Value"=w207:bool)  [unwired: 2 in, 2 out]
                  n250 = property on="As gas Flow" class="DigNum (strict)"() -> ("Value"=w208:dbl)  [unwired: 2 in, 2 out]
                  n251 = And(x=w206, y=w207) -> (x .and. y?=w205:bool)
                  n252 = call "set_As_gas.vi"("Active"=w209, "As_Gas Flow"=w208, "Gas In"=w209, "Run"=w205) -> ()  [unwired: 12 in]
                }
              }
            }
            frame True {
            }
          }
        }
        frame #5 {
          n253 = case shown="False" w210 {
            frame False {
              n254 = property on="P liq?" class="Bool (strict)"() -> ("Value"=w211:bool)  [unwired: 2 in, 2 out]
              n255 = case shown="True" w211 {
                frame False {
                  w212 = FALSE ("As_Gas Active")
                  n256 = call "set_P_Liq.vi"("flow 1"=0.0 ("As_Gas Flow"), "Remote"=w212, "Run"=w212, "Bubbler In"=w212, "Active"=w212) -> ()  [unwired: 5 in]
                }
                frame True {
                  w218 = TRUE ("As_Gas Active")
                  n257 = property on="Prep P liq" class="Bool (strict)"() -> ("Value"=w215:bool)  [unwired: 2 in, 2 out]
                  n258 = property on="Run P Liq" class="Bool (strict)"() -> ("Value"=w216:bool)  [unwired: 2 in, 2 out]
                  n259 = property on="P Liq Flow" class="DigNum (strict)"() -> ("Value"=w217:dbl)  [unwired: 2 in, 2 out]
                  n260 = And(x=w215, y=w216) -> (x .and. y?=w214:bool)
                  n261 = call "set_P_Liq.vi"("flow 1"=w217, "Run"=w214, "Bubbler In"=w218, "Active"=w218) -> ()  [unwired: 6 in]
                }
              }
            }
            frame True {
            }
          }
        }
      }
    }
    frame "Run" {
      n262 = stacked-sequence {
        tunnel: w222 -> [_ w227 _ _]
        tunnel: w219 -> [w224 _ _ w290]
        tunnel: [_ _ _ w289] -> w221
        tunnel: w220 -> [_ _ _ w291]
        frame #0 {
          n263 = call "Get_Argument.vi"("Argument"="run_started", "Argument List"=w224) -> ("Enabled"=w223:bool)
          n264 = local write "run started"(w223) -> ()
        }
        frame #1 {
          n265 = property on="prep_time" class="DigNum (strict)"() -> ("Value"=w228:dbl)  [unwired: 2 in, 2 out]
          n266 = Greater Or Equal?(x=w227, y=w228) -> (x >= y?=w226:bool)
          n267 = local write "prep_done"(w226) -> ()
        }
        frame #2 {
          n268 = local read "run started"() -> (w230:bool)
          n269 = Not(x=w230) -> (.not. x?=w229:bool)
          n270 = stacked-sequence {
            tunnel: w229 -> [w232 w236 w245 w254 w263 w272 w283]
            frame #0 {
              n271 = case shown="True" w232 {
                tunnel: ["run: " "pre-run: "] -> w231
                frame False {
                }
                frame True {
                }
              }
              n272 = property on="Status Out" class="Str"("Value"=w231) -> ()  [unwired: 2 in, 2 out]
            }
            frame #1 {
              n273 = property on="Status Out" class="Str"() -> ("Value"=w242:string)  [unwired: 2 in, 2 out]
              n274 = property on="Al?" class="Bool (strict)"() -> ("Value"=w243:bool)  [unwired: 2 in, 2 out]
              n275 = property on="Run Al" class="Bool (strict)"() -> ("Value"=w235:bool)  [unwired: 2 in, 2 out]
              n276 = property on="Prep Al" class="Bool (strict)"() -> ("Value"=w237:bool)  [unwired: 2 in, 2 out]
              n277 = call "flow_strings.vi"("string in"=w242, "is first in?"=TRUE, "use source?"=w243, "name"="Al", "run source?"=w235, "prep source?"=w237, "is prep?"=w236) -> ("string out"=w241:string, "is first out?"=w240:bool)
              n278 = property on="Status Out" class="Str"("Value"=w241) -> ()  [unwired: 2 in, 2 out]
              n279 = property on="first" class="Bool (strict)"("Value"=w240) -> ()  [unwired: 2 in, 2 out]
            }
            frame #2 {
              n280 = property on="first" class="Bool (strict)"() -> ("Value"=w248:bool)  [unwired: 2 in, 2 out]
              n281 = property on="Status Out" class="Str"() -> ("Value"=w251:string)  [unwired: 2 in, 2 out]
              n282 = property on="Ga?" class="Bool (strict)"() -> ("Value"=w249:bool)  [unwired: 2 in, 2 out]
              n283 = property on="Run Ga" class="Bool (strict)"() -> ("Value"=w244:bool)  [unwired: 2 in, 2 out]
              n284 = property on="Prep Ga" class="Bool (strict)"() -> ("Value"=w246:bool)  [unwired: 2 in, 2 out]
              n285 = call "flow_strings.vi"("string in"=w251, "is first in?"=w248, "use source?"=w249, "name"="Ga", "run source?"=w244, "prep source?"=w246, "is prep?"=w245) -> ("string out"=w252:string, "is first out?"=w247:bool)
              n286 = property on="Status Out" class="Str"("Value"=w252) -> ()  [unwired: 2 in, 2 out]
              n287 = property on="first" class="Bool (strict)"("Value"=w247) -> ()  [unwired: 2 in, 2 out]
            }
            frame #3 {
              n288 = property on="first" class="Bool (strict)"() -> ("Value"=w258:bool)  [unwired: 2 in, 2 out]
              n289 = property on="Status Out" class="Str"() -> ("Value"=w260:string)  [unwired: 2 in, 2 out]
              n290 = property on="In?" class="Bool (strict)"() -> ("Value"=w261:bool)  [unwired: 2 in, 2 out]
              n291 = property on="Run In" class="Bool (strict)"() -> ("Value"=w253:bool)  [unwired: 2 in, 2 out]
              n292 = property on="Prep In" class="Bool (strict)"() -> ("Value"=w255:bool)  [unwired: 2 in, 2 out]
              n293 = call "flow_strings.vi"("string in"=w260, "is first in?"=w258, "use source?"=w261, "name"="In", "run source?"=w253, "prep source?"=w255, "is prep?"=w254) -> ("string out"=w257:string, "is first out?"=w256:bool)
              n294 = property on="Status Out" class="Str"("Value"=w257) -> ()  [unwired: 2 in, 2 out]
              n295 = property on="first" class="Bool (strict)"("Value"=w256) -> ()  [unwired: 2 in, 2 out]
            }
            frame #4 {
              n296 = property on="first" class="Bool (strict)"() -> ("Value"=w266:bool)  [unwired: 2 in, 2 out]
              n297 = property on="Status Out" class="Str"() -> ("Value"=w268:string)  [unwired: 2 in, 2 out]
              n298 = property on="PH3?" class="Bool (strict)"() -> ("Value"=w269:bool)  [unwired: 2 in, 2 out]
              n299 = property on="Run P gas" class="Bool (strict)"() -> ("Value"=w262:bool)  [unwired: 2 in, 2 out]
              n300 = property on="Prep P gas" class="Bool (strict)"() -> ("Value"=w264:bool)  [unwired: 2 in, 2 out]
              n301 = call "flow_strings.vi"("string in"=w268, "is first in?"=w266, "use source?"=w269, "name"="PH3", "run source?"=w262, "prep source?"=w264, "is prep?"=w263) -> ("string out"=w267:string, "is first out?"=w265:bool)
              n302 = property on="Status Out" class="Str"("Value"=w267) -> ()  [unwired: 2 in, 2 out]
              n303 = property on="first" class="Bool (strict)"("Value"=w265) -> ()  [unwired: 2 in, 2 out]
            }
            frame #5 {
              n304 = property on="first" class="Bool (strict)"() -> ("Value"=w275:bool)  [unwired: 2 in, 2 out]
              n305 = property on="Status Out" class="Str"() -> ("Value"=w277:string)  [unwired: 2 in, 2 out]
              n306 = property on="AsH3?" class="Bool (strict)"() -> ("Value"=w278:bool)  [unwired: 2 in, 2 out]
              n307 = property on="Run As gas" class="Bool (strict)"() -> ("Value"=w271:bool)  [unwired: 2 in, 2 out]
              n308 = property on="Prep As gas" class="Bool (strict)"() -> ("Value"=w273:bool)  [unwired: 2 in, 2 out]
              n309 = call "flow_strings.vi"("string in"=w277, "is first in?"=w275, "use source?"=w278, "name"="AsH3", "run source?"=w271, "prep source?"=w273, "is prep?"=w272) -> ("string out"=w274:string, "is first out?"=w276:bool)
              n310 = property on="Status Out" class="Str"("Value"=w274) -> ()  [unwired: 2 in, 2 out]
              n311 = property on="first" class="Bool (strict)"("Value"=w276) -> ()  [unwired: 2 in, 2 out]
            }
            frame #6 {
              n312 = property on="P liq?" class="Bool (strict)"() -> ("Value"=w282:bool)  [unwired: 2 in, 2 out]
              n313 = property on="Run P Liq" class="Bool (strict)"() -> ("Value"=w281:bool)  [unwired: 2 in, 2 out]
              n314 = property on="first" class="Bool (strict)"() -> ("Value"=w286:bool)  [unwired: 2 in, 2 out]
              n315 = property on="Status Out" class="Str"() -> ("Value"=w288:string)  [unwired: 2 in, 2 out]
              n316 = property on="Prep P liq" class="Bool (strict)"() -> ("Value"=w280:bool)  [unwired: 2 in, 2 out]
              n317 = call "flow_strings.vi"("string in"=w288, "is first in?"=w286, "use source?"=w282, "name"="P liq", "run source?"=w281, "prep source?"=w280, "is prep?"=w283) -> ("string out"=w285:string, "is first out?"=w284:bool)
              n318 = property on="Status Out" class="Str"("Value"=w285) -> ()  [unwired: 2 in, 2 out]
              n319 = property on="first" class="Bool (strict)"("Value"=w284) -> ()  [unwired: 2 in, 2 out]
            }
          }
        }
        frame #3 {
          n320 = local read "run started"() -> (w294:bool)
          n321 = local read "prep_done"() -> (w292:bool)
          n322 = Not(x=w294) -> (.not. x?=w295:bool)
          n323 = And(x=w292, y=w295) -> (x .and. y?=w293:bool)
          n324 = stacked-sequence {
            tunnel: w293 -> [w299]
            tunnel: w291 -> [w298]
            tunnel: w290 -> [w297]
            tunnel: [w296] -> w289
            frame #0 {
              n325 = case shown="True" w299 {
                tunnel: w298 -> [_ w303]
                tunnel: w297 -> [w300 w302]
                tunnel: [w300 w301] -> w296
                frame False {
                }
                frame True {
                  n326 = stacked-sequence {
                    tunnel: w303 -> [w304 w311 w321 w328 w335 _ w346 w353]
                    tunnel: w302 -> [_ _ _ _ _ w343 _ _]
                    tunnel: [_ _ _ _ _ w342 _ _] -> w301
                    frame #0 {
                      n327 = case shown="False" w304 {
                        frame False {
                          n328 = property on="Al?" class="Bool (strict)"() -> ("Value"=w305:bool)  [unwired: 2 in, 2 out]
                          n329 = case shown="True" w305 {
                            frame False {
                              w306 = FALSE ("Al Active")
                              n330 = call "set_Al.vi"("ALMFC1"=0.0 ("Aluminum Flow"), "Remote"=w306, "Run"=w306, "Bubbler In"=w306, "Active"=w306) -> ()  [unwired: 5 out]
                            }
                            frame True {
                              w310 = TRUE ("Al Active")
                              n331 = property on="Al Flow" class="DigNum (strict)"() -> ("Value"=w309:dbl)  [unwired: 2 in, 2 out]
                              n332 = property on="Run Al" class="Bool (strict)"() -> ("Value"=w308:bool)  [unwired: 2 in, 2 out]
                              n333 = call "set_Al.vi"("ALMFC1"=w309, "Run"=w308, "Bubbler In"=w310, "Active"=w310) -> ()  [unwired: 1 in, 5 out]
                            }
                          }
                        }
                        frame True {
                        }
                      }
                    }
                    frame #1 {
                      n334 = case shown="False" w311 {
                        frame False {
                          n335 = property on="Ga?" class="Bool (strict)"() -> ("Value"=w312:bool)  [unwired: 2 in, 2 out]
                          n336 = case shown="True" w312 {
                            frame False {
                              w314 = FALSE ("Ga Active")
                              w313 = 0.0 ("Ga Flow 1")
                              n337 = call "set_Ga.vi"("Active"=w314, "GAMFC3"=w313, "GAMFC2"=w313, "GAMFC1"=w313, "Bubbler In"=w314, "H2 Dilute"=w314, "Run"=w314, "Remote"=w314) -> ()  [unwired: 8 out]
                            }
                            frame True {
                              w319 = TRUE ("Ga Active")
                              n338 = property on="GAMFC3 var" class="DigNum (strict)"() -> ("Value"=w315:dbl)  [unwired: 2 in, 2 out]
                              n339 = property on="Ga Dilution" class="Bool (strict)"() -> ("Value"=w318:bool)  [unwired: 2 in, 2 out]
                              n340 = property on="Run Ga" class="Bool (strict)"() -> ("Value"=w320:bool)  [unwired: 2 in, 2 out]
                              n341 = property on="GAMFC2 var" class="DigNum (strict)"() -> ("Value"=w316:dbl)  [unwired: 2 in, 2 out]
                              n342 = property on="GAMFC1 var" class="DigNum (strict)"() -> ("Value"=w317:dbl)  [unwired: 2 in, 2 out]
                              n343 = call "set_Ga.vi"("Active"=w319, "GAMFC3"=w315, "GAMFC2"=w316, "GAMFC1"=w317, "Bubbler In"=w319, "H2 Dilute"=w318, "Run"=w320, "Remote"=w319) -> ()  [unwired: 8 in]
                            }
                          }
                        }
                        frame True {
                        }
                      }
                    }
                    frame #2 {
                      n344 = case shown="False" w321 {
                        frame False {
                          n345 = property on="In?" class="Bool (strict)"() -> ("Value"=w322:bool)  [unwired: 2 in, 2 out]
                          n346 = case shown="True" w322 {
                            frame False {
                              w324 = FALSE ("In Remote")
                              n347 = call "set_In.vi"("INMFC1"=0.0 ("Indium Flow"), "Remote"=w324, "Run"=w324, "Bubbler In"=w324, "Active"=w324) -> ()  [unwired: 5 out]
                            }
                            frame True {
                              w327 = TRUE ("In Run")
                              n348 = property on="Run In" class="Bool (strict)"() -> ("Value"=w325:bool)  [unwired: 2 in, 2 out]
                              n349 = property on="In Flow" class="DigNum (strict)"() -> ("Value"=w326:dbl)  [unwired: 2 in, 2 out]
                              n350 = call "set_In.vi"("INMFC1"=w326, "Run"=w325, "Bubbler In"=w327, "Active"=w327) -> ()  [unwired: 1 in, 5 out]
                            }
                          }
                        }
                        frame True {
                        }
                      }
                    }
                    frame #3 {
                      n351 = case shown="False" w328 {
                        frame False {
                          n352 = property on="PH3?" class="Bool (strict)"() -> ("Value"=w329:bool)  [unwired: 2 in, 2 out]
                          n353 = case shown="True" w329 {
                            frame False {
                              w330 = FALSE ("P_Gas Active")
                              n354 = call "set_P_gas.vi"("Run"=w330, "Gas In"=w330, "Active"=w330, "P_Gas Remote"=w330, "H2 Flush"=w330, "P_Gas Flow"=0.0) -> ()
                            }
                            frame True {
                              w334 = TRUE ("P_Gas Active")
                              n355 = property on="P gas Flow" class="DigNum (strict)"() -> ("Value"=w333:dbl)  [unwired: 2 in, 2 out]
                              n356 = property on="Run P gas" class="Bool (strict)"() -> ("Value"=w332:bool)  [unwired: 2 in, 2 out]
                              n357 = call "set_P_gas.vi"("Active"=w334, "P_Gas Remote"=w332, "H2 Flush"=w334, "P_Gas Flow"=w333) -> ()  [unwired: 2 in]
                            }
                          }
                        }
                        frame True {
                        }
                      }
                    }
                    frame #4 {
                      n358 = case shown="False" w335 {
                        frame False {
                          n359 = property on="AsH3?" class="Bool (strict)"() -> ("Value"=w336:bool)  [unwired: 2 in, 2 out]
                          n360 = case shown="True" w336 {
                            frame False {
                              w337 = FALSE ("As_Gas Active")
                              n361 = call "set_As_gas.vi"("Active"=w337, "As_Gas Flow"=0.0, "Gas In"=w337, "H2 Flush"=w337, "Run"=w337, "Remote"=w337) -> ()  [unwired: 10 in]
                            }
                            frame True {
                              w340 = TRUE ("As_Gas Active")
                              n362 = property on="Run As gas" class="Bool (strict)"() -> ("Value"=w339:bool)  [unwired: 2 in, 2 out]
                              n363 = property on="As gas Flow" class="DigNum (strict)"() -> ("Value"=w341:dbl)  [unwired: 2 in, 2 out]
                              n364 = call "set_As_gas.vi"("Active"=w340, "As_Gas Flow"=w341, "Gas In"=w340, "Run"=w339) -> ()  [unwired: 12 in]
                            }
                          }
                        }
                        frame True {
                        }
                      }
                    }
                    frame #5 {
                      n365 = call "Set_Argument.vi"("Enable"=TRUE, "Argument"="run_started", "Argument List In"=w343) -> ("Argument List Out"=w342:string[])
                    }
                    frame #6 {
                      n366 = case shown="False" w346 {
                        frame False {
                          n367 = property on="P liq?" class="Bool (strict)"() -> ("Value"=w347:bool)  [unwired: 2 in, 2 out]
                          n368 = case shown="False" w347 {
                            frame False {
                              w349 = FALSE ("In Remote")
                              n369 = call "set_P_Liq.vi"("flow 1"=0.0 ("Indium Flow"), "Remote"=w349, "Run"=w349, "Bubbler In"=w349, "Active"=w349) -> ()  [unwired: 5 in]
                            }
                            frame True {
                              w352 = TRUE ("In Run")
                              n370 = property on="P Liq Flow" class="DigNum (strict)"() -> ("Value"=w351:dbl)  [unwired: 2 in, 2 out]
                              n371 = property on="Run P Liq" class="Bool (strict)"() -> ("Value"=w350:bool)  [unwired: 2 in, 2 out]
                              n372 = call "set_P_Liq.vi"("flow 1"=w351, "Run"=w350, "Bubbler In"=w352, "Active"=w352) -> ()  [unwired: 6 in]
                            }
                          }
                        }
                        frame True {
                        }
                      }
                    }
                    frame #7 {
                      n373 = case shown="False" w353 {
                        frame False {
                          n374 = property on="P liq?" class="Bool (strict)"() -> ("Value"=w354:bool)  [unwired: 2 in, 2 out]
                          n375 = case shown="False" w354 {
                            frame False {
                              w356 = FALSE ("In Remote")
                              n376 = call "set_P_Liq.vi"("flow 1"=0.0 ("Indium Flow"), "Remote"=w356, "Run"=w356, "Bubbler In"=w356, "Active"=w356) -> ()  [unwired: 5 in]
                            }
                            frame True {
                              w359 = TRUE ("In Run")
                              n377 = property on="P Liq Flow" class="DigNum (strict)"() -> ("Value"=w358:dbl)  [unwired: 2 in, 2 out]
                              n378 = property on="Run P Liq" class="Bool (strict)"() -> ("Value"=w357:bool)  [unwired: 2 in, 2 out]
                              n379 = call "set_P_Liq.vi"("flow 1"=w358, "Run"=w357, "Bubbler In"=w359, "Active"=w359) -> ()  [unwired: 6 in]
                            }
                          }
                        }
                        frame True {
                        }
                      }
                    }
                  }
                }
              }
            }
          }
        }
      }
    }
    frame "End" {
    }
    frame "Idle" {
    }
  }
  "Argument List Out" <- w10
